vi "Read CAN FIFO Direct Dispatch.vi"(8 "error in (no error)":errorcluster, 9 "Timeout (ms)":i32, 11 "CIFTag in":refnum<class "CIFChannels.lvclass">) -> (0 "error out":errorcluster, 1 "timed out?":bool, 2 "Data":u8[](array[numeric]) format="%.0x", 3 "CIFTag out":refnum<class "CIF_NIChn_FifoCAN.lvclass">, 4 "Header":T1)   [LabVIEW 2021, in "CIF_NIChn_FifoCAN.lvclass"]
uses:
  CIF_NIChn_FifoCAN.lvclass
  CIF_NIChn_FifoCAN.lvclass/CIF_NIChn_FifoCAN.ctl
  CIFChannels/Typedef/Direction.ctl
  CIFChannels/CIFChannels.lvclass
  CIFChannels/Typedef/Channel State.ctl
  NIChn/CIF_NIChn.lvclass
  D:/dev/Packages/Channel_Manager/src/CIF_NIChn/NIChn/CIF_NIChn.lvclass
  D:/dev/Packages/Channel_Manager/src/CIFChannels/CIFChannels.lvclass
  D:/dev/Packages/Channel_Manager/src/CIF_NIChn/FIFO_CAN/CIF_NIChn_FifoCAN.lvclass
  <vilib>/CIFChannels/CIFChannelCore.lvlib
  ChannelCommon/typedef/FIFO Header.ctl
  ChannelCommon/ChannelCommon.lvlib
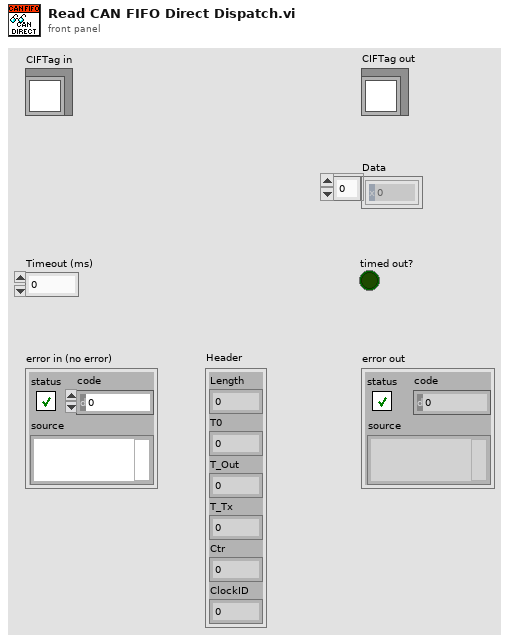
[diagram p1: front panel]
types:
  T1 = typedef "ChannelCommon.lvlib/FIFO Header.ctl" = cluster{"Length":u64, "T0":i64, "T_Out":i64, "T_Tx":i64, "Ctr":u64, "ClockID":u8}
  T2 = typedef "CIFChannels.lvclass/Channel State.ctl" = enum16{"Creating", "Disconnected", "Connecting", "Connected", "Destroyed"}
  T3 = typedef "CIFChannels.lvclass/Direction.ctl" = enum16{"Publisher", "Subscriber"}
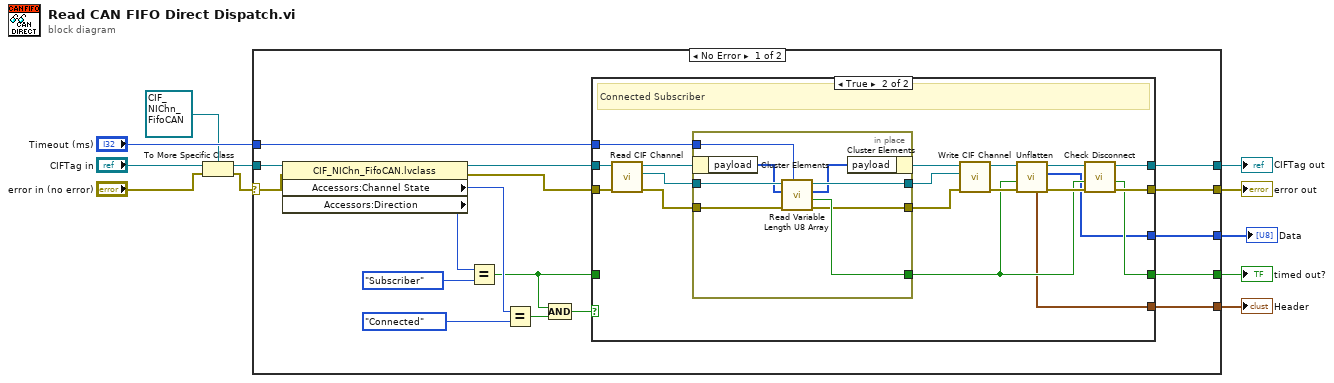
[diagram p0: block diagram]
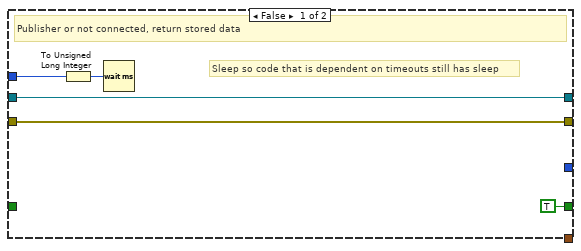
[diagram p2: hidden frame]
diagram:
  n1 = To More Specific Class(target class=refnum<class "CIF_NIChn_FifoCAN.lvclass"> refnum ("CIFTag in"), reference="CIFTag in", error in="error in (no error)") -> (specific class reference=w4:refnum<class "CIF_NIChn_FifoCAN.lvclass">, error out=w3:errorcluster)
  n2 = case shown="No Error" w3 {
    selector: w3 -> [w26 w62]
    tunnel: [w15 w62] -> w11
    tunnel: [w16 w61] -> w10
    tunnel: w4 -> [w27 w61]
    tunnel: [w28 _] -> w9
    tunnel: "Timeout (ms)" -> [w14 _]
    tunnel: [w13 _] -> w7
    tunnel: [w12 _] -> w1
    frame No Error {
      n3 = property class="CIF_NIChn_FifoCAN.lvclass"(reference=w27, error in=w26) -> (reference out=w25:refnum<class "CIF_NIChn_FifoCAN.lvclass">, error out=w24:errorcluster, "Accessors:Channel State"=w21:T2, "Accessors:Direction"=w23:T3)
      n4 = Equal?(x=w23, y=Direction."Subscriber") -> (x = y?=w17:bool)
      n5 = Equal?(x=w21, y=Channel_State."Connected") -> (x = y?=w19:bool)
      n6 = Compound Arithmetic op=AND(w17, w19) -> (w18:bool)
      n7 = case shown="True" w18 {
        tunnel: [TRUE ("timeout out") w42] -> w28
        tunnel: w24 -> [w32 w51]
        tunnel: w25 -> [w33 w52]
        tunnel: w17 -> [_ _]
        tunnel: [w33 w50] -> w16
        tunnel: [w32 w49] -> w15
        tunnel: w14 -> [w29 w41]
        tunnel: [_ w35] -> w13
        tunnel: [_ w34] -> w12
        frame False {
          # "Sleep so code that is dependent on timeouts still has sleep"
          # "Publisher or not connected, return stored data"
          n8 = To Unsigned Long Integer(number=w29) -> (unsigned 32bit integer=w30:u32)
          n9 = Wait (ms)(milliseconds to wait=w30) -> ()  [unwired: 1 out]
        }
        frame True {
          # "Connected Subscriber"
          n10 = call "Read CIF Channel.vi"("error in (no error)"=w51, "CIFTag in"=w52) -> ("error out"=w46:errorcluster, "CIF Channel"=w47:refnum<k21>, "CIFTag out"=w48:refnum<class "CIF_NIChn_FifoCAN.lvclass">)  [unwired: 7 in]
          n11 = in-place {
            in-place-border: [w58] -> w36
            in-place-border: w47 -> [w60]
            in-place-border: w46 -> [w59]
            in-place-border: [w57] -> w43
            in-place-border: [w56] -> w44
            in-place-border: w41 -> [w55]
            n12 = in-place-cluster #1(w48) -> ("payload"=w54:u8[])
            n13 = call <vilib>:"Read Variable Length U8 Array.vi"("Timeout (ms)"=w55, "error in"=w59, "Payload in"=w54, "CIF Channel in"=w60) -> ("error out"=w56:errorcluster, "Timed out?"=w58:bool, "Payload out"=w53:u8[], "CIF Channel out"=w57:refnum<k21>)  [unwired: 4 in]
            n14 = in-place-cluster #1("payload"=w53) -> (w45:refnum<class "CIF_NIChn_FifoCAN.lvclass">)
          }
          n15 = call "Write CIF Channel.vi"("error in (no error)"=w44, "CIF Channel"=w43, "CIFTag in"=w45) -> ("error out"=w39:errorcluster, "CIFTag out"=w40:refnum<class "CIF_NIChn_FifoCAN.lvclass">)  [unwired: 7 in]
          n16 = call "Unflatten.vi"("error in (no error)"=w39, "timeout in"=w36, "CIFFifoCAN in"=w40) -> ("error out"=w37:errorcluster, "Data"=w34:u8[], "CIFFifoCAN out"=w38:refnum<class "CIF_NIChn_FifoCAN.lvclass">, "Header"=w35:T1)  [unwired: 5 in]
          n17 = call "Check Disconnect.vi"("error in (no error)"=w37, "timeout in"=w36, "CIFTag in"=w38) -> ("error out"=w49:errorcluster, "timeout out"=w42:bool, "CIFTag out"=w50:refnum<class "CIF_NIChn_FifoCAN.lvclass">)  [unwired: 5 in, 1 out]
        }
      }
    }
    frame Error {
    }
  }
  "error out" <- w11
  "CIFTag out" <- w10
  "timed out?" <- w9
  "Header" <- w7
  "Data" <- w1
